vi "Acquire.vi"(7 "Qbus":refnum<class "Qbus.lvclass">, 8 "error in (no error)":errorcluster, 11 "config":T1={"active cameras"=[], "poll interval (sec)"=1.0}) -> (0 "error out":errorcluster, 1 "error cameras":T2[](array[typedef]), 2 "new data":T6[](array[typedef]), 3 "config out":T1={"active cameras"=[], "poll interval (sec)"=1.0}, 4 "error text":string[](array[string]))   [LabVIEW 2017, in "IrAcquisition.lvlib"]
uses:
  <vilib>/addons/InsightCM/Devices/Shared/Ir/IrAcquisition/IrAcquisition.lvlib
  <vilib>/addons/InsightCM/Devices/Shared/Common/DataFlow/controls/Data.ctl
  <vilib>/addons/InsightCM/Utilities/DataAccessors/controls/wfmSGL_DVR.ctl
  <vilib>/addons/PointValueMap/controls/PointMap.ctl
  <vilib>/addons/InsightCM/Devices/Shared/Common/DataFlow/controls/Type.ctl
  <vilib>/addons/InsightCM/Devices/Shared/Ir/IrAcquisition/controls/camera.ctl
  <vilib>/userdefined/High Color/IMAQdx.ctl
  <vilib>/vision/Image Controls.llb/IMAQ Image.ctl
  <vilib>/addons/InsightCM/Devices/Shared/Ir/IrAcquisition/controls/config.ctl
  <vilib>/addons/Qbus/Qbus.lvclass
  InsightCM/Devices/WebServices/Ir/DataAccessors/action.ctl
  <vilib>/addons/PointValueMap/subVIs/Point_Write_string.vi
  <vilib>/vision/driver/NI_Vision_Acquisition_Software.lvlib
  <vilib>/addons/PointValueMap/PointValueMap.lvlib
  <vilib>/addons/InsightCM/Devices/Shared/Common/DataFlow/DataFlow.lvlib
  InsightCM/Devices/WebServices/Ir/DataAccessors/VisionWebServiceData.lvlib
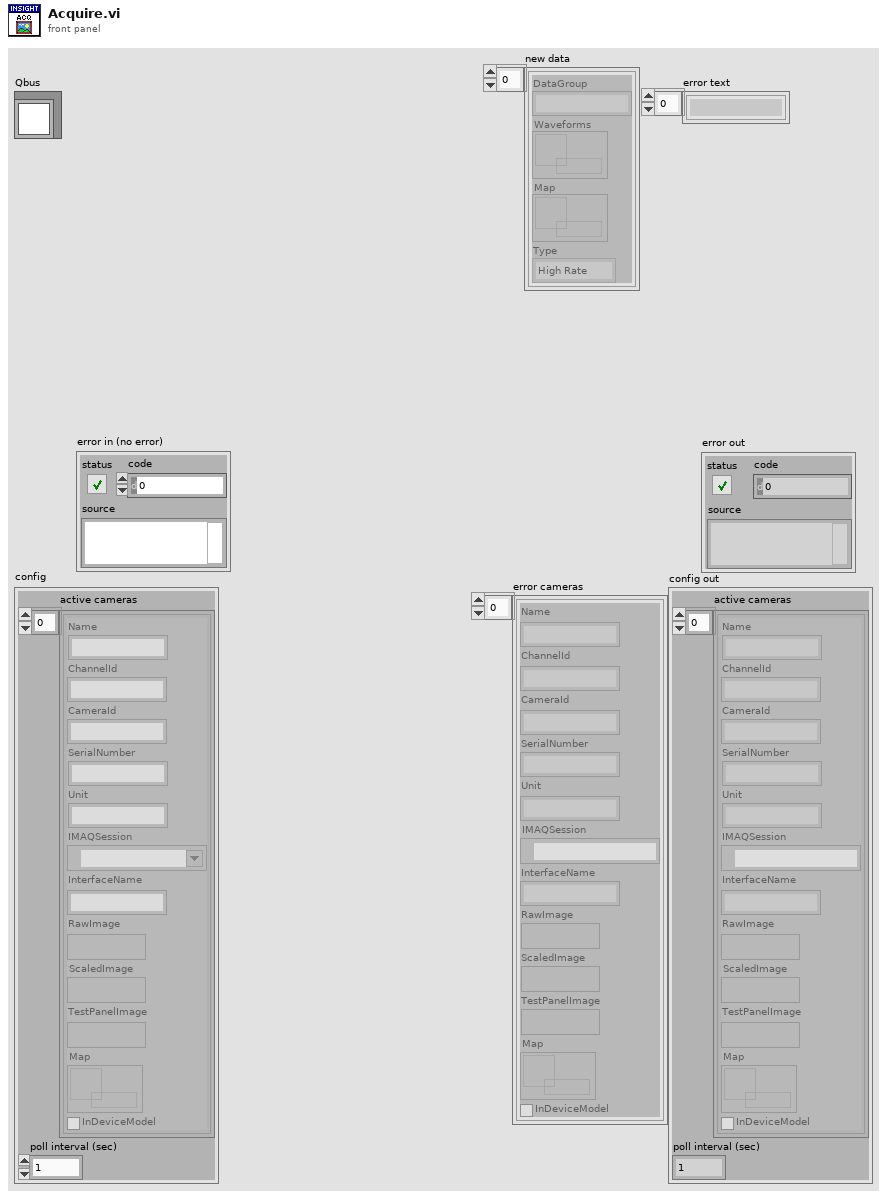
[diagram p1: front panel]
types:
  T1 = typedef "IrAcquisition.lvlib/config.ctl" = cluster{"active cameras":T2[], "poll interval (sec)":dbl}
  T2 = typedef "IrAcquisition.lvlib/camera.ctl" = cluster{"Name":string, "ChannelId":string, "CameraId":string, "SerialNumber":string, "Unit":string, "IMAQSession":T3, "InterfaceName":string, "RawImage":T4, "ScaledImage":T4, "TestPanelImage":T4, "Map":T5, "InDeviceModel":bool}
  T3 = typedef "IMAQdx.ctl" = refnum<k21>
  T4 = typedef "IMAQ Image.ctl" = refnum<image>
  T5 = typedef "PointValueMap.lvlib/PointMap.ctl" = refnum<data-value>
  T6 = typedef "DataFlow.lvlib/Data.ctl" = cluster{"DataGroup":string, "Waveforms":T7, "Map":T5, "Type":T8}
  T7 = typedef "wfmSGL_DVR.ctl" = refnum<data-value>
  T8 = typedef "DataFlow.lvlib/Type.ctl" = enum16{"High Rate", "Low Rate", "Burst Mode"}
  T9 = typedef "VisionWebServiceData.lvlib/action.ctl" = enum16{"Get", "Set"}
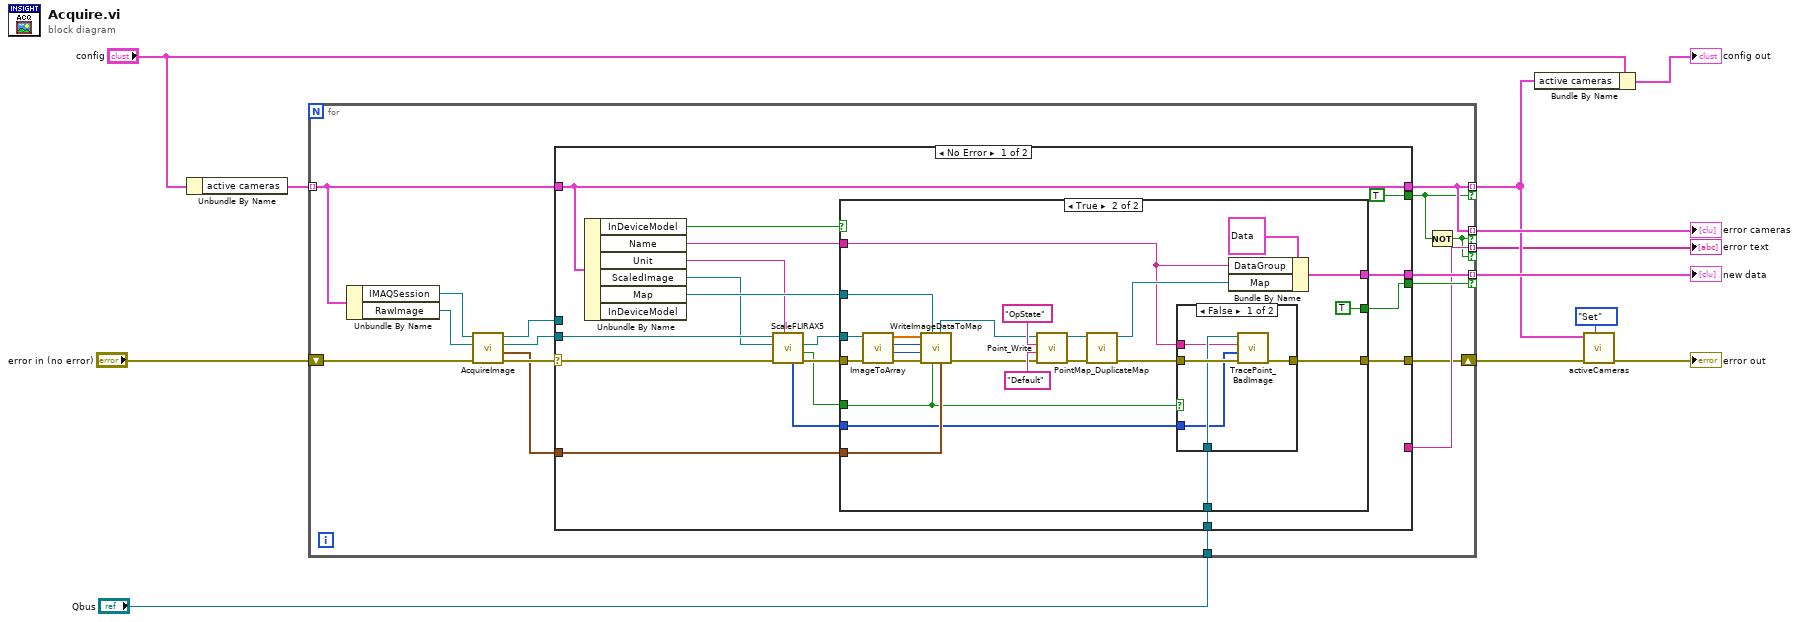
[diagram p0: block diagram]
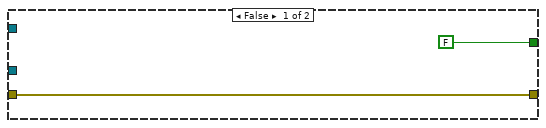
[diagram p2: hidden frame]
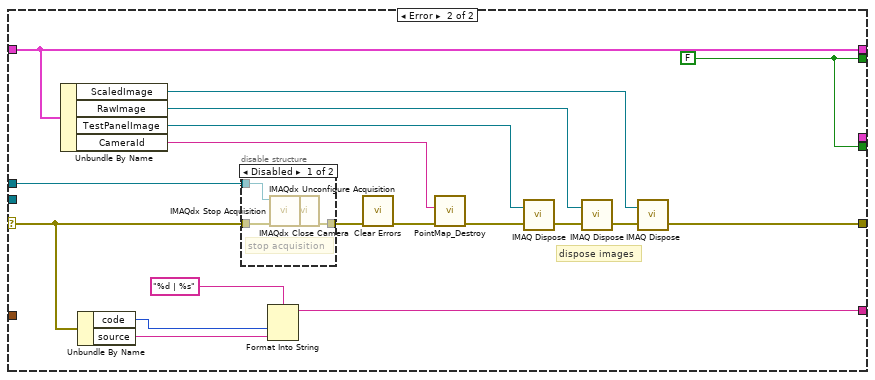
[diagram p4: hidden frame]
diagram:
  n1 = Unbundle By Name("config") -> ("active cameras"=w8:T2[])
  n2 = for {
    tunnel: w8 -> [w20] mode=indexing
    tunnel: [w19] -> w10 mode=indexing if=w15
    tunnel: [w22] -> w11 mode=indexing if=w17
    tunnel: [w19] -> w6 mode=indexing if=w18
    shift-right: [w14] -> w4
    shift-left: "error in (no error)" -> [w28]
    tunnel: [w16] -> w2 mode=indexing if=w15
    tunnel: "Qbus" -> [w13]
    n3 = Unbundle By Name(w20) -> ("IMAQSession"=w27:T3, "RawImage"=w23:T4)
    n4 = call <vilib>:"AcquireImage.vi"("error in (no error)"=w28, "image in"=w23, "session in"=w27) -> ("error out"=w26:errorcluster, "timestamp"=w21:timestamp, "image out"=w24:T4, "session out"=w25:T3)  [unwired: 5 in]
    n5 = case shown="No Error" w26 {
      selector: w26 -> [w34 w83]
      tunnel: [w41 w93] -> w14
      tunnel: w25 -> [_ w95]
      tunnel: w24 -> [w36 _]
      tunnel: [w45 _] -> w22
      tunnel: [TRUE w84] -> w18
      tunnel: w21 -> [w44 _]
      tunnel: w20 -> [w42 w85]
      tunnel: [w42 w85] -> w19
      tunnel: [w37 w84] -> w17
      tunnel: [_ w80] -> w16
      tunnel: w13 -> [w40 _]
      frame No Error {
        n6 = Unbundle By Name(w42) -> ("InDeviceModel"=w38:bool, "Name"=w39:string, "Unit"=w29:string, "ScaledImage"=w35:T4, "Map"=w43:T5)  [unwired: 1 out]
        n7 = call <vilib>:"ScaleFLIRAX5.vi"("unit"=w29, "error in (no error)"=w34, "ScaledImage"=w35, "RawImage"=w36) -> ("error out"=w33:errorcluster, "image ok"=w31:bool, "ScaledImage"=w30:T4, "histogram"=w32:u32[])  [unwired: 4 in]
        n8 = case shown="True" w38 {
          tunnel: w33 -> [w47 w49]
          tunnel: [_ w71] -> w45
          tunnel: w44 -> [_ w55]
          tunnel: w43 -> [_ w59]
          tunnel: [w47 w64] -> w41
          tunnel: w40 -> [_ w63]
          tunnel: w39 -> [_ w62]
          tunnel: [FALSE TRUE] -> w37
          tunnel: w32 -> [_ w52]
          tunnel: w31 -> [_ w51]
          tunnel: w30 -> [_ w50]
          frame False {
          }
          frame True {
            n9 = call <vilib>:"ImageToArray.vi"("error in (no error)"=w49, "image"=w50) -> ("error out"=w60:errorcluster, "height"=w56:i32, "width"=w57:i32, "image data"=w58:sgl[])  [unwired: 6 in]
            n10 = call <vilib>:"WriteImageDataToMap.vi"("image timestamp"=w55, "image status"=w51, "map"=w59, "error in (no error)"=w60, "image height"=w56, "image width"=w57, "image data"=w58) -> ("error out"=w53:errorcluster, "map out"=w54:T5)  [unwired: 3 in]
            n11 = call-poly <vilib>:"Point_Write.vi"("Error In"=w53, "Value"="Default", "Tag"="OpState", "Map"=w54) -> ("Error Out"=w69:errorcluster, "Map Out"=w68:T5)  [unwired: 6 in]
            n12 = call <vilib>:"PointMap_DuplicateMap.vi"("error in (no error)"=w69, "map in"=w68) -> ("error out"=w65:errorcluster, "duplicate map"=w70:T5)  [unwired: 8 in]
            n13 = case shown="False" w51 {
              tunnel: w65 -> [w77 w78]
              tunnel: [w76 w78] -> w64
              tunnel: w63 -> [w75 _]
              tunnel: w62 -> [w74 _]
              tunnel: w52 -> [w73 _]
              frame False {
                n14 = call <vilib>:"TracePoint_BadImage.vi"("error in (no error)"=w77, "histogram"=w73, "Camera"=w74, "Qbus"=w75) -> ("error out"=w76:errorcluster)  [unwired: 7 in]
              }
              frame True {
              }
            }
            n15 = Bundle By Name(cluster=T6 {"DataGroup"="", "Waveforms"=refnum, "Map"=refnum, "Type"=enum."High Rate"} ("data"), "DataGroup"=w62, "Map"=w70) -> (w71:T6)
          }
        }
      }
      frame Error {
        w84 = FALSE
        # "dispose images"
        n16 = Unbundle By Name(w85) -> ("ScaledImage"=w91:T4, "RawImage"=w90:T4, "TestPanelImage"=w86:T4, "CameraId"=w89:string)
        n17 = Unbundle By Name(w83) -> ("code"=w81:i32, "source"=w79:string)
        n18 = disable-structure shown="Disabled" {
          disable-tunnel: [w99 w104] -> w96
          disable-tunnel: w83 -> [w98 w104]
          disable-tunnel: w95 -> [w97 _]
          frame Disabled {
            # "stop acquisition"
            n19 = call <vilib>:"IMAQdx Stop Acquisition.vi"("error in"=w98, "Session In"=w97) -> ("error out"=w100:errorcluster, "Session Out"=w101:T3)  [unwired: 8 out]
            n20 = call <vilib>:"IMAQdx Unconfigure Acquisition.vi"("error in"=w100, "Session In"=w101) -> ("error out"=w103:errorcluster, "Session Out"=w102:T3)  [unwired: 8 out]
            n21 = call <vilib>:"IMAQdx Close Camera.vi"("error in"=w103, "Session In"=w102) -> ("error out"=w99:errorcluster)  [unwired: 9 out]
          }
          frame Enabled {
            # "simulated"
          }
        }
        n22 = Format Into String(format string="%d | %s", w81, w79) -> (resulting string=w80:string)  [unwired: 2 in, 1 out]
        n23 = call <vilib>:"Clear Errors.vi"("error in (no error)"=w96) -> ("error out"=w92:errorcluster)  [unwired: 5 in, 1 out]
        n24 = call <vilib>:"PointMap_Destroy.vi"("error in (no error)"=w92, "Name"=w89) -> ("error out"=w88:errorcluster)  [unwired: 9 in]
        n25 = call "IMAQ Dispose"("Image"=w86, "error in (no error)"=w88) -> ("error out"=w87:errorcluster)  [unwired: 4 in]
        n26 = call "IMAQ Dispose"("Image"=w90, "error in (no error)"=w87) -> ("error out"=w94:errorcluster)  [unwired: 4 in]
        n27 = call "IMAQ Dispose"("Image"=w91, "error in (no error)"=w94) -> ("error out"=w93:errorcluster)  [unwired: 4 in]
      }
    }
    n28 = Not(x=w18) -> (.not. x?=w15:bool)
  }
  "new data" <- w11
  "error cameras" <- w10
  "error text" <- w2
  n29 = Bundle By Name(cluster="config", "active cameras"=w6) -> (→"config out":T1)
  n30 = call "activeCameras.vi"("action"=action."Set", "error in (no error)"=w4, "cameras"=w6) -> ("error out"=→"error out":errorcluster)  [unwired: 7 in, 1 out]
